vi "Remove Attribute - One.vi"(8 "error in (no error)":errorcluster, 10 "Attribute":string, 11 "YAML Parser in":refnum<class "YAML Parser.lvclass">) -> (0 "error out":errorcluster, 2 "found":bool, 3 "YAML Parser out":refnum<class "YAML Parser.lvclass">)   [LabVIEW 2015, in "YAML Parser.lvclass"]
uses:
  YAML Parser.lvclass
  YAML Parser.lvclass/YAML Parser.ctl
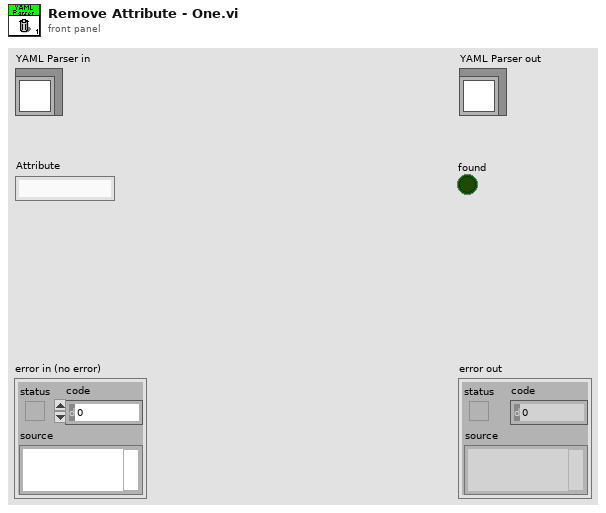
[diagram p1: front panel]
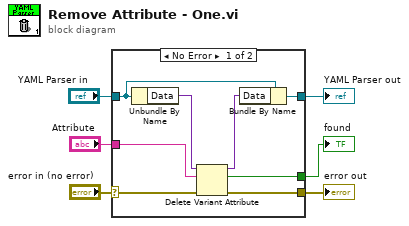
[diagram p0: block diagram]
diagram:
  n1 = case shown="No Error" "error in (no error)" {
    selector: "error in (no error)" -> [w10 w16]
    tunnel: [w9 w16] -> w5
    tunnel: [w13 w15] -> w3
    tunnel: "YAML Parser in" -> [w14 w15]
    tunnel: "Attribute" -> [w11 _]
    tunnel: [w7 _] -> w1
    frame No Error {
      n2 = Unbundle By Name(w14) -> ("Data"=w12:variant)
      n3 = Delete Variant Attribute(4:w10, 6:w11, 7:w12) -> (0:w9:errorcluster, 2:w7:bool, 3:w8:variant)
      n4 = Bundle By Name(cluster=w14, "Data"=w8) -> (w13:refnum<class "YAML Parser.lvclass">)
    }
    frame Error {
    }
  }
  "error out" <- w5
  "YAML Parser out" <- w3
  "found" <- w1
